vi "Load_Template_Globals.vi"(1 "Non Blank Channels":i32[](array[numeric]), 2 "Channel Names":string[](array[string]), 3 "Template-read":path) -> (0 "Valid Template File?":bool)   [LabVIEW 2020]
uses:
  Data plotting/subVIs/Dispose_Channel.ctl
  Controls/Global_mode.ctl
  Results_plotter_Global.vi
panel:
  in  "Dispose":T1
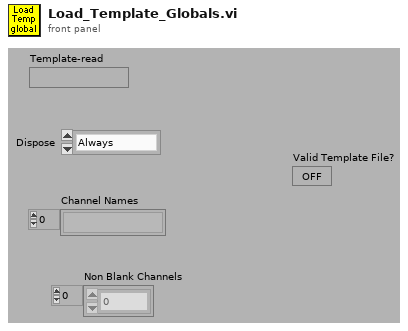
[diagram p1: front panel]
types:
  T1 = typedef "Dispose_Channel.ctl" = enum16{"Always", "If Blank", "Never"}
  T2 = typedef "Global_mode.ctl" = enum16{"Read Global", "Load Global From File", "Write Global to File"}
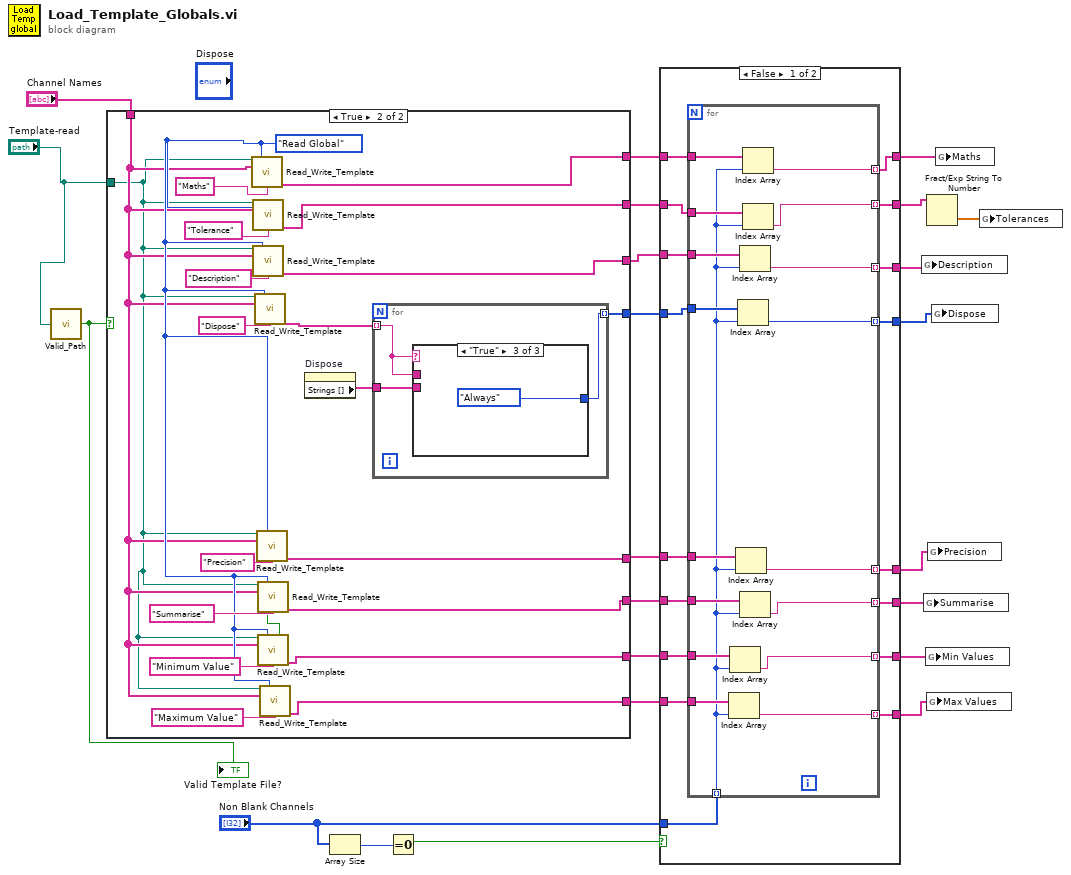
[diagram p0: block diagram]
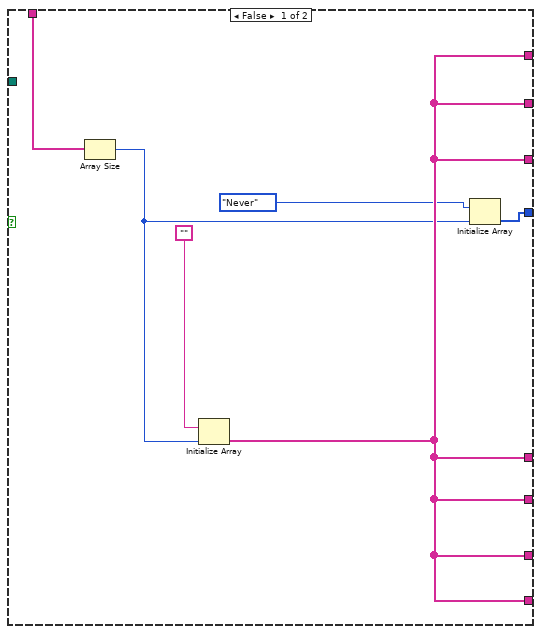
[diagram p3: hidden frame]
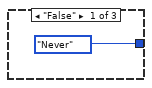
[diagram p4: hidden frame]
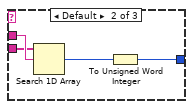
[diagram p5: hidden frame]
diagram:
  n1 = call "Valid_Path.vi"("Filename"="Template-read") -> ("Valid Path?"=w21:bool)
  "Valid Template File?" <- w21
  n2 = case shown="True" w21 {
    tunnel: "Template-read" -> [_ w35]
    tunnel: "Channel Names" -> [w28 w36]
    tunnel: [w27 w46] -> w16
    tunnel: [w27 w45] -> w15
    tunnel: [w26 w31] -> w14
    tunnel: [w27 w44] -> w13
    tunnel: [w27 w43] -> w12
    tunnel: [w27 w41] -> w20
    tunnel: [w27 w34] -> w17
    tunnel: [w27 w33] -> w18
    frame False {
      n3 = Array Size(array=w28) -> (size(s)=w25:i32)
      n4 = Initialize Array("", w25) -> (w27:string[])
      n5 = Initialize Array(Dispose_Channel."Never" ("Dispose"), w25) -> (w26:T1[])
    }
    frame True {
      w37 = Global_mode."Read Global" ("Mode")
      n6 = call "Read_Write_Template.vi"("Template File"=w35, "Mode"=w37, "Channel names In"=w36, "Data type"="Maths") -> ("1D Info Out"=w41:string[])  [unwired: 4 in, 7 out]
      n7 = call "Read_Write_Template.vi"("Template File"=w35, "Mode"=w37, "Channel names In"=w36, "Data type"="Tolerance") -> ("1D Info Out"=w43:string[])  [unwired: 4 in, 7 out]
      n8 = call "Read_Write_Template.vi"("Template File"=w35, "Mode"=w37, "Channel names In"=w36, "Data type"="Description") -> ("1D Info Out"=w44:string[])  [unwired: 4 in, 7 out]
      n9 = call "Read_Write_Template.vi"("Template File"=w35, "Mode"=w37, "Channel names In"=w36, "Data type"="Dispose") -> ("1D Info Out"=w32:string[])  [unwired: 4 in, 7 out]
      n10 = call "Read_Write_Template.vi"("Template File"=w35, "Mode"=w37, "Channel names In"=w36, "Data type"="Precision") -> ("1D Info Out"=w45:string[])  [unwired: 4 in, 7 out]
      n11 = call "Read_Write_Template.vi"("Template File"=w35, "Mode"=w37, "Channel names In"=w36, "Data type"="Minimum Value") -> ("Freshly Loaded?"=w39:bool, "1D Info Out"=w34:string[])  [unwired: 4 in, 6 out]
      n12 = call "Read_Write_Template.vi"("Template File"=w35, "Mode"=w37, "Channel names In"=w36, "Save file"=w39, "Data type"="Summarise") -> ("1D Info Out"=w46:string[])  [unwired: 3 in, 7 out]
      n13 = call "Read_Write_Template.vi"("Template File"=w35, "Mode"=w37, "Channel names In"=w36, "Data type"="Maximum Value") -> ("1D Info Out"=w33:string[])  [unwired: 4 in, 7 out]
      n14 = property on="Dispose" class="Enum (strict)"() -> ("Strings []"=w30:string[])  [unwired: 2 in, 2 out]
      n15 = for {
        tunnel: w32 -> [w54] mode=indexing
        tunnel: [w52] -> w31 mode=indexing
        tunnel: w30 -> [w53]
        n16 = case shown="\"True\"" w54 {
          tunnel: w54 -> [_ w59 _]
          tunnel: w53 -> [_ w58 _]
          tunnel: [Dispose_Channel."Never" ("Dispose") w56 Dispose_Channel."Always" ("Dispose")] -> w52
          frame "False" {
          }
          frame Default {
            n17 = Search 1D Array(1D array=w58, element=w59) -> (index of element=w57:i32)  [unwired: 1 in]
            n18 = To Unsigned Word Integer(number=w57) -> (unsigned 16bit integer=w56:u16)
          }
          frame "True" {
          }
        }
      }
    }
  }
  n19 = Array Size(array="Non Blank Channels") -> (size(s)=w4:i32)
  n20 = Equal To 0?(x=w4) -> (x = 0?=w3:bool)
  n21 = case shown="False" w3 {
    tunnel: w20 -> [w77 w102]
    tunnel: [w76 w102] -> w19
    tunnel: w18 -> [w75 w95]
    tunnel: w17 -> [w74 w96]
    tunnel: w16 -> [w73 w97]
    tunnel: w15 -> [w72 w98]
    tunnel: w14 -> [w71 w99]
    tunnel: w13 -> [w70 w100]
    tunnel: w12 -> [w69 w101]
    tunnel: [w68 w101] -> w2
    tunnel: [w67 w100] -> w11
    tunnel: [w66 w99] -> w10
    tunnel: [w65 w98] -> w9
    tunnel: [w64 w97] -> w8
    tunnel: [w63 w96] -> w7
    tunnel: [w62 w95] -> w6
    tunnel: "Non Blank Channels" -> [w61 _]
    frame False {
      n22 = for {
        tunnel: w77 -> [w94]
        tunnel: w61 -> [w78] mode=indexing
        tunnel: [w93] -> w76 mode=indexing
        tunnel: w69 -> [w92]
        tunnel: w70 -> [w91]
        tunnel: w71 -> [w90]
        tunnel: w72 -> [w89]
        tunnel: w73 -> [w88]
        tunnel: w74 -> [w87]
        tunnel: w75 -> [w86]
        tunnel: [w85] -> w68 mode=indexing
        tunnel: [w84] -> w67 mode=indexing
        tunnel: [w83] -> w66 mode=indexing
        tunnel: [w82] -> w65 mode=indexing
        tunnel: [w81] -> w64 mode=indexing
        tunnel: [w80] -> w63 mode=indexing
        tunnel: [w79] -> w62 mode=indexing
        n23 = Index Array(array=w86, index=w78) -> (element=w79:string)
        n24 = Index Array(array=w87, index=w78) -> (element=w80:string)
        n25 = Index Array(array=w89, index=w78) -> (element=w82:string)
        n26 = Index Array(array=w90, index=w78) -> (element=w83:u16)
        n27 = Index Array(array=w91, index=w78) -> (element=w84:string)
        n28 = Index Array(array=w88, index=w78) -> (element=w81:string)
        n29 = Index Array(array=w94, index=w78) -> (element=w93:string)
        n30 = Index Array(array=w92, index=w78) -> (element=w85:string)
      }
    }
    frame True {
    }
  }
  n31 = global write "Results_plotter_Global.vi" "Description"(w11) -> ()
  n32 = global write "Results_plotter_Global.vi" "Summarise"(w8) -> ()
  n33 = global write "Results_plotter_Global.vi" "Min Values"(w7) -> ()
  n34 = Fract/Exp String To Number(string=w2) -> (number=w1:dbl[])  [unwired: 4 out]
  n35 = global write "Results_plotter_Global.vi" "Max Values"(w6) -> ()
  n36 = global write "Results_plotter_Global.vi" "Precision"(w9) -> ()
  n37 = global write "Results_plotter_Global.vi" "Dispose"(w10) -> ()
  n38 = global write "Results_plotter_Global.vi" "Maths"(w19) -> ()
  n39 = global write "Results_plotter_Global.vi" "Tolerances"(w1) -> ()
